vi "Write TDMS.vi"(4 "Append Index":i32, 6 "Commands":string, 8 "error in (no error)":errorcluster, 9 "Notes":string, 10 "Data (Dictionary)":T1[](array[typedef]), 11 "path":path) -> (0 "error out":errorcluster, 3 "path out":path)   [LabVIEW 2016, in "LV-Data.TDMS.lvclass"]
uses:
  LV-Data.TDMS.lvclass
  LV-Data/Typedefs/Dictionary--cluster.ctl
  LV-Data/LV-Data.lvclass
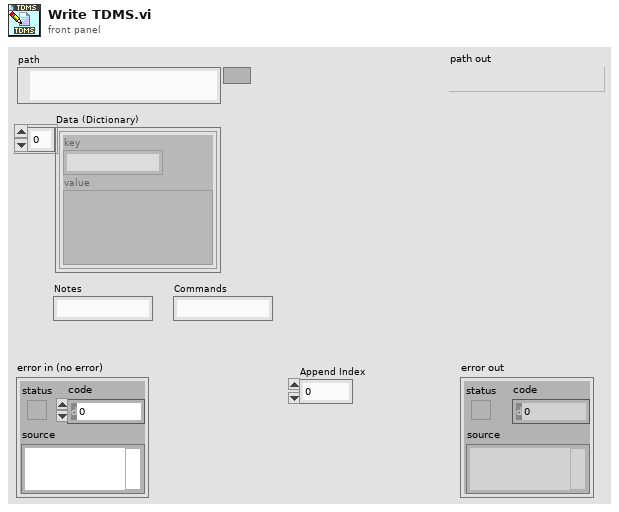
[diagram p1: front panel]
types:
  T1 = typedef "LV-Data.lvclass/Dictionary--cluster.ctl" = cluster{"key":string, "value":variant}
  T2 = enum16{"open", "open or create", "create or replace", "create", "open (read-only)"}
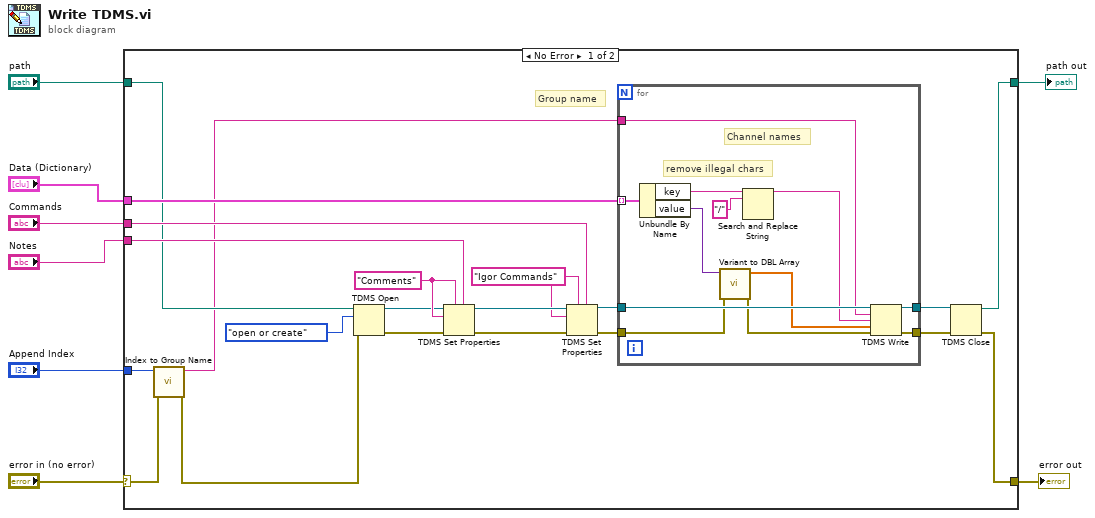
[diagram p0: block diagram]
diagram:
  n1 = case shown="No Error" "error in (no error)" {
    selector: "error in (no error)" -> [w10 w43]
    tunnel: [w18 w43] -> w4
    tunnel: "Append Index" -> [w12 _]
    tunnel: "path" -> [w15 w42]
    tunnel: "Notes" -> [w21 _]
    tunnel: "Commands" -> [w22 _]
    tunnel: "Data (Dictionary)" -> [w23 _]
    tunnel: [w14 w42] -> w5
    frame No Error {
      w25 = "Igor Commands" ("attrib name")
      w24 = "Comments" ("attrib name")
      # "Group name"
      n2 = call "Index to Group Name.vi"("error in (no error)"=w10, "Append Index"=w12) -> ("error out"=w11:errorcluster, "group name in (Untitled)"=w9:string)  [unwired: 8 in]
      n3 = TDMS Open(8:w11, 10:T2."open or create" ("operation (0:open)"), 11:w15) -> (0:w20:errorcluster, 3:w16:refnum<k34>)  [unwired: 4 in]
      n4 = TDMS Set Properties(5:w21, 7:w24, 8:w20, 10:w24, 11:w16) -> (0:w28:errorcluster, 3:w29:refnum<k34>)  [unwired: 1 in, 2 out]
      n5 = TDMS Set Properties(5:w22, 7:w25, 8:w28, 10:w25, 11:w29) -> (0:w27:errorcluster, 3:w26:refnum<k34>)  [unwired: 1 in, 2 out]
      n6 = for {
        tunnel: w23 -> [w36] mode=indexing
        tunnel: w27 -> [w33]
        tunnel: w26 -> [w40]
        tunnel: [w39] -> w19
        tunnel: [w38] -> w17
        tunnel: w9 -> [w30]
        # "Channel names"
        # "remove illegal chars"
        n7 = Unbundle By Name(w36) -> ("key"=w37:string, "value"=w32:variant)
        n8 = call "Variant to DBL Array.vi"("error in (no error)"=w33, "Data (Variant)"=w32) -> ("error out"=w34:errorcluster, "1D Array"=w31:dbl[])  [unwired: 7 in, 1 out]
        n9 = Search and Replace String(input string=w37, search string="/") -> (result string=w35:string)  [unwired: 6 in, 3 out]
        n10 = TDMS Write(0:w40, 5:w30, 7:w35, 9:w31, 11:w34) -> (4:w38:refnum<k34>, 15:w39:errorcluster)  [unwired: 1 in, 2 out]
      }
      n11 = TDMS Close(8:w19, 11:w17) -> (0:w18:errorcluster, 3:w14:path)
    }
    frame Error {
    }
  }
  "error out" <- w4
  "path out" <- w5
